vi "mqttCmdBuildVarHdr.vi"(0 "mqttConnect in":refnum<class "mqttCmdConnect.lvclass">, 11 "error in (no error)":errorcluster) -> (4 "mqttConnect out":refnum<class "mqttCmdConnect.lvclass">, 8 "varHeader":u8[](array[numeric]) format="%x", 15 "error out":errorcluster)   [LabVIEW 2019, in "mqttCmdConnect.lvclass"]
uses:
  mqttCmdConnect.lvclass
  mqttCmdConnect.lvclass/mqttCmdConnect.ctl
  mqtt.lvclass/mqtt.ctl
  mqtt.lvclass
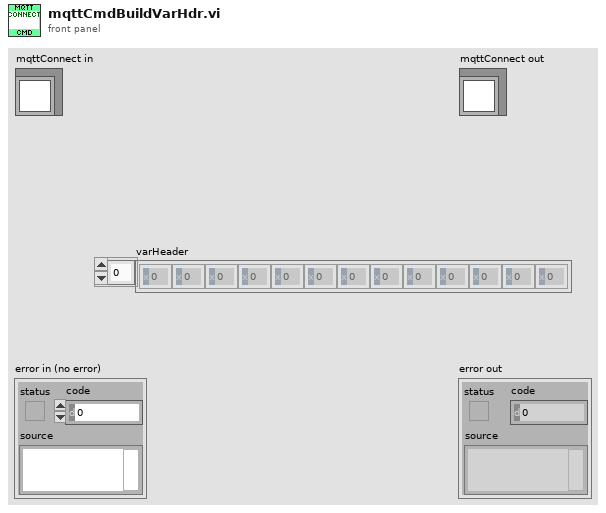
[diagram p1: front panel]
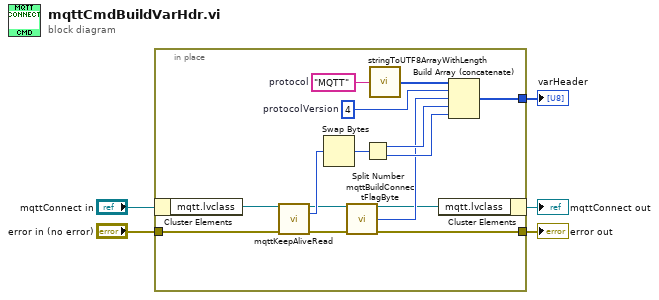
[diagram p0: block diagram]
diagram:
  n1 = in-place {
    in-place-border: [w13] -> w5
    in-place-border: "error in (no error)" -> [w11]
    in-place-border: [w8] -> w3
    w17 = u8 4  # protocolVersion
    w15 = "MQTT"  # protocol
    n2 = in-place-cluster #1("mqttConnect in") -> ("mqtt.lvclass"=w7:refnum<class "mqtt.lvclass">)
    n3 = call "mqttKeepAliveRead.vi"("mqtt in"=w7, "error in (no error)"=w11) -> ("mqtt out"=w10:refnum<class "mqtt.lvclass">, "keepAlive(sec)"=w12:u16, "error out"=w9:errorcluster)  [unwired: 11 in]
    n4 = Swap Bytes(anything=w12) -> (byte swapped=w20:u16)
    n5 = call "mqttBuildConnectFlagByte.vi"("mqtt in"=w10, "error in (no error)"=w9) -> ("mqtt out"=w6:refnum<class "mqtt.lvclass">, "connFlagByte out"=w16:u8, "error out"=w8:errorcluster)  [unwired: 11 in]
    n6 = Split Number(x=w20) -> (hi(x)=w19:u8, lo(x)=w18:u8)
    n7 = call "stringToUTF8ArrayWithLength.vi"("string"=w15) -> ("UTF8[]"=w14:u8[])  [unwired: 14 in]
    n8 = in-place-cluster #1("mqtt.lvclass"=w6) -> (→"mqttConnect out":refnum<class "mqttCmdConnect.lvclass">)
    n9 = Build Array (concatenate)(w14, w17, w16, w19, w18) -> (w13:u8[])
  }
  "error out" <- w3
  "varHeader" <- w5
